vi "Fpga-FIXParser-TestHarness.vi"   [LabVIEW 2020]
uses:
  Common/Fpga-Field.Value.ctl
  <vilib>/Platform/TimedLoop/XDataNode/timing_clust.ctl
  <vilib>/Platform/TimedLoop/XDataNode/nitl_modes.ctl
  <vilib>/Platform/TimedLoop/XDataNode/wakeup.ctl
  <vilib>/rvi/Emulation/niFpgaSctlEmulationGetInTimedLoop.vi
  <vilib>/rvi/Emulation/niFpgaEmulationReportErrorSimple.vi
  <vilib>/rvi/Emulation/niFpgaGetClockAttributes.vi
  <vilib>/rvi/Emulation/niFpgaCriticalErrorInLSC.vi
  <vilib>/rvi/interface/RandomDataEmulation/niFpgaRandomDataHandleErrors.vi
  <vilib>/rvi/Emulation/niFpgaEmulationIsFPGAContextNoSignature.vi
  <vilib>/rvi/errors/niFpgaSetErrorForExecOnDevCompSimple.vi
  <vilib>/rvi/eio/common/nirviEmuReportErrorAndStop.vi
  <vilib>/rvi/DataTransferAndStorage/Container/Common/niFpgaContainerGetUniqueNameForEmu.vi
  <vilib>/rvi/FIFO/Fifo_Resource/nirvififoEmulationSetSize.vi
  <vilib>/rvi/FIFO/Fifo_Resource/nirviFifoEmulationQueueMgr.vi
  <instcachedir>/0/nirviFifoEmulationQueueMgr_E5CAEC123FF24DC58D834DCA3CDAA9B5.lvgen/nirviFifoEmulationQueueMgr_E5CAEC123FF24DC58D834DCA3CDAA9B5_002.vi
  <vilib>/rvi/FIFO/Fifo_Resource/nirvififoEmulationDetermineInputValidOut.vi
  <vilib>/rvi/FIFO/Fifo_Resource/nirvififoEmulationCreateLock.vi
  <vilib>/rvi/Emulation/niFpgaProcessEmulError.vi
  <vilib>/rvi/FIFO/Fifo_Resource/nirvififoEmulationObtainLock.vi
  <vilib>/rvi/FIFO/Fifo_Resource/nirvififoEmulationReleaseLock.vi
  <vilib>/rvi/occurrence/nirviWaitOnOccurrenceBase.vi
  <vilib>/rvi/errors/nirviReportUnexpectedCaseInternalError.vi
  <vilib>/rvi/errors/nirviReportUnexpectedCaseInternalError (U32).vi
  <instcachedir>/0/nirviFifoEmulationQueueMgr_E5CAEC123FF24DC58D834DCA3CDAA9B5.lvgen/nirviFifoEmulationQueueMgr_E5CAEC123FF24DC58D834DCA3CDAA9B5_012.vi
  <vilib>/Utility/error.llb/Clear Errors.vi
  <vilib>/Platform/TimedLoop/XDataNode/XDataNode.xnode
  <vilib>/rvi/DataTransferAndStorage/Container/XNode/niFpgaContainer.xnode
  <vilib>/rvi/interface/RandomDataEmulation/nirviRandomDataFpgaReadWriteTemplate.vi
  <vilib>/rvi/FIFO/Fifo_Resource/nirvififoEmulationWrite.vi
  <vilib>/rvi/FIFO/Fifo_Resource/nirvififoEmulationRead.vi
  <vilib>/Platform/TimedLoop/XDataNode/XDNodeRunTimeDep.lvlib
types:
  T1 = typedef "Fpga-Field.Value.ctl" = cluster{"Field.Num":u16, "Int.Value":u16, "Str.Value":u8[], "Date.Value":u64, "Str.Length":u8}
  T2 = typedef "XDNodeRunTimeDep.lvlib/timing_clust.ctl" = cluster{"Expected End [f-1]":u64, "Actual End [f-1]":u64, "Finished Late? [f-1]":bool, "Expected End [i-1]":u64, "Actual End [i-1]":u64, "Finished Late? [i-1]":bool, "Expected Start [i]":u64, "Actual Start [i]":u64, "Expected Start [f]":u64, "Actual Start [f]":u64, "Source Name":string, "Structure Name":string, "Period":i64, "Deadline":i64, "Offset":i64, "Start":i64, "Priority":i32, "Timeout":i32, "Mode":T3, "Wakeup Reason":T4, "Error":errorcluster, "Source Type":string, "Secondary Source Type":string, "Global End Time":u64, "Global Start Time":u64, "Frame Duration":u64, "Iteration Duration":u64, "Assigned CPU":i32, "I/O Scan Engine Mode":u32}
  T3 = typedef "XDNodeRunTimeDep.lvlib/nitl_modes.ctl" = enum32{"No Change", "Process missed periods, maintain original phase", "Discard missed periods, maintain original phase", "Process missed periods, ignore original phase", "Discard missed periods, ignore original phase"}
  T4 = typedef "XDNodeRunTimeDep.lvlib/wakeup.ctl" = enum32{"Normal", "Aborted", "Asynchronous wakeup", "Timing source error", "Timed loop error", "Timeout"}
  T5 = cluster{"Field.Num":u16, "Int.Value":u16, "Str.Value":u8[], "Date.Value":u64, "Str.Length":u8}
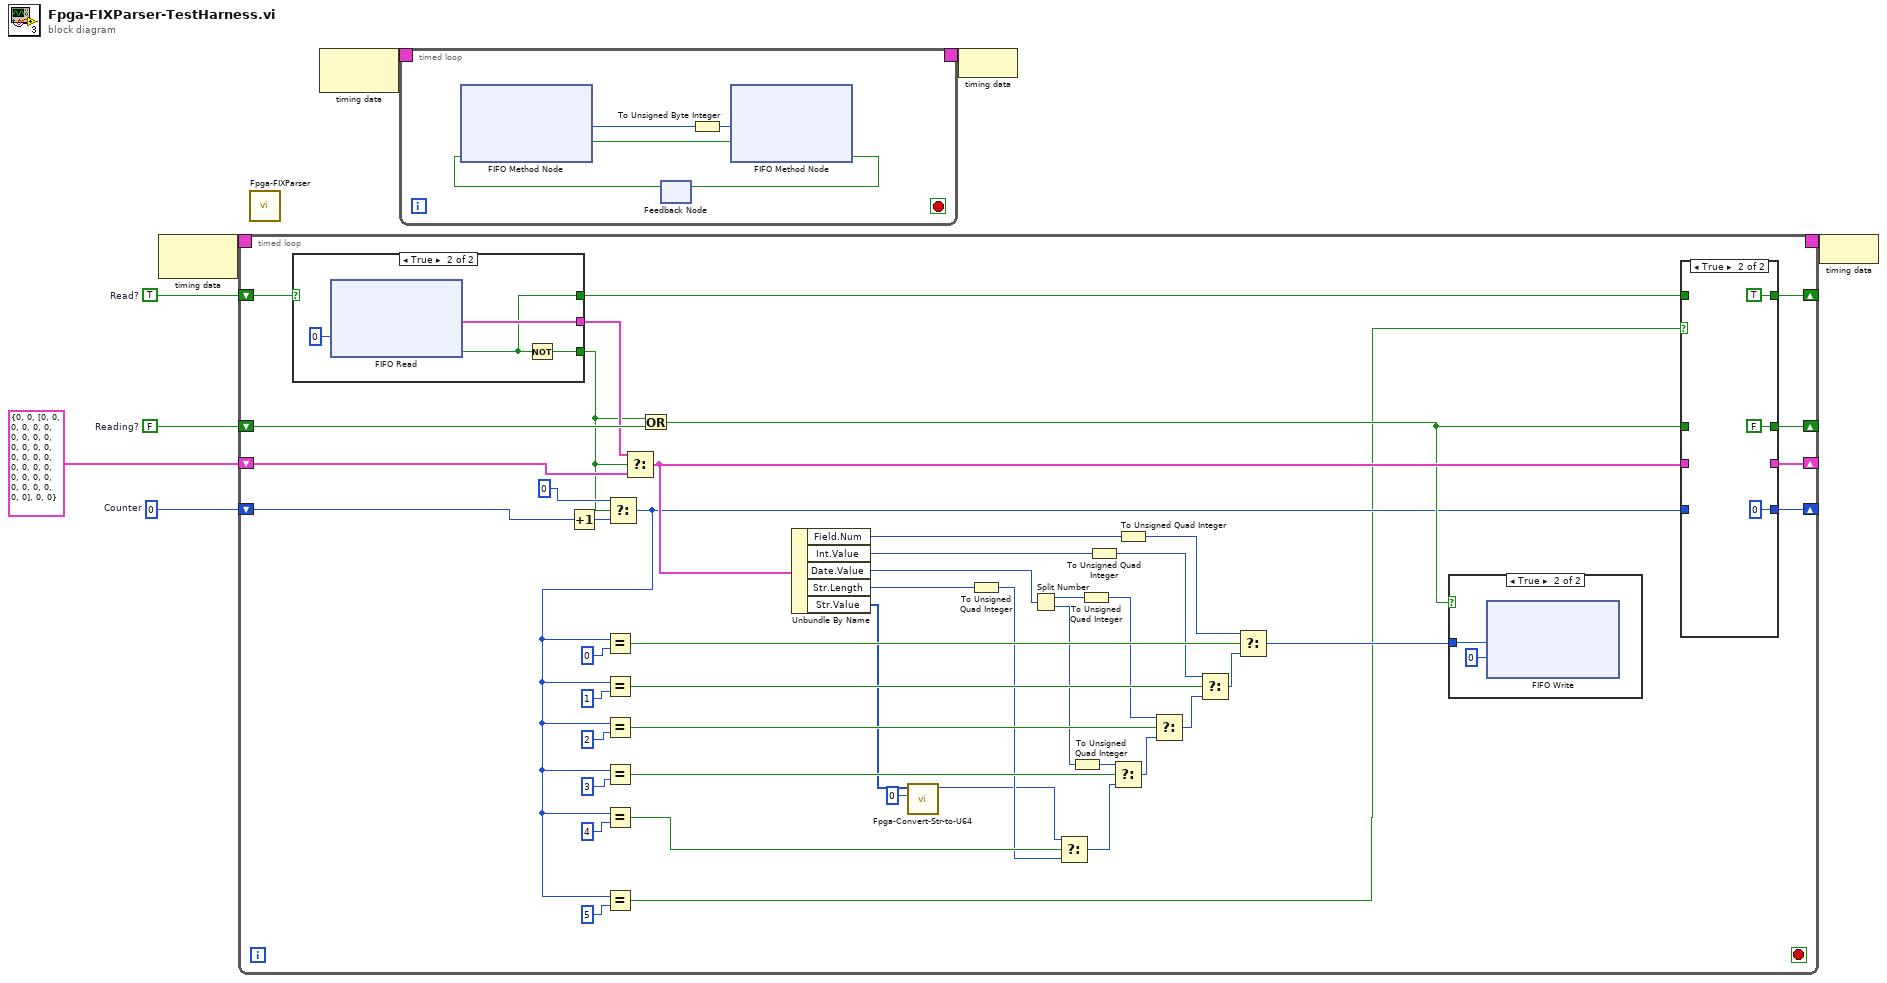
[diagram p0: block diagram]
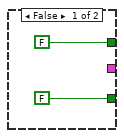
[diagram p4: hidden frame]
diagram:
  w2 = FALSE  # Reading?
  w3 = i16 0  # Counter
  w4 = TRUE  # Read?
  n1 = node-c288() -> (w6:T2)  [unwired: 1 in]
  n2 = timed-loop {
    timing: w6 -> [_]
    timing-out: [_] -> w5
    shift-right: [w53] -> _
    shift-left: w4 -> [w54]
    shift-right: [w51] -> _
    shift-left: w3 -> [w39]
    shift-right: [w49] -> _
    shift-left: w2 -> [w50]
    shift-right: [w34] -> _
    shift-left: T1 {"Field.Num"=0, "Int.Value"=0, "Str.Value"=[0, 0, 0, 0, 0, 0, 0, 0, 0, 0, 0, 0, 0, 0, 0, 0, 0, 0, 0, 0, 0, 0, 0, 0, 0, 0, 0, 0, 0, 0, 0, 0], "Date.Value"=0, "Str.Length"=0} ("Field.Value.Pair") -> [w32]
    stop <- _ stop-if-true
    n3 = case shown="True" w54 {
      tunnel: [_ w69] -> w47
      tunnel: [FALSE ("Timed Out?") w68] -> w31
      tunnel: [FALSE w67] -> w52
      frame False {
      }
      frame True {
        n4 = xnode ("FIFO Read")("Timeout"=0) -> ("Element"=w69:T5, "Timed Out?"=w67:bool)  [unwired: 1 in, 1 out]
        n5 = Not(x=w67) -> (.not. x?=w68:bool)
      }
    }
    n6 = Increment(x=w39) -> (x+1=w55:i16)
    n7 = Select(t=i16 0, s=w31, f=w55) -> (s? t:f=w17:i16)
    n8 = Equal?(x=w17, y=i16 0) -> (x = y?=w43:bool)
    n9 = Equal?(x=w17, y=i16 1) -> (x = y?=w41:bool)
    n10 = Equal?(x=w17, y=i16 2) -> (x = y?=w37:bool)
    n11 = Equal?(x=w17, y=i16 3) -> (x = y?=w21:bool)
    n12 = Equal?(x=w17, y=i16 4) -> (x = y?=w15:bool)
    n13 = Equal?(x=w17, y=i16 5) -> (x = y?=w16:bool)
    n14 = Select(t=w47, s=w31, f=w32) -> (s? t:f=w33:T1)
    n15 = Or(x=w31, y=w50) -> (x .or. y?=w30:bool)
    n16 = Unbundle By Name(w33) -> ("Field.Num"=w28:u16, "Int.Value"=w27:u16, "Date.Value"=w26:u64, "Str.Length"=w9:u8, "Str.Value"=w12:u8[])
    n17 = call "Fpga-Convert-Str-to-U64.vi"("startingIndex"=0, "Str.Value"=w12) -> ("Numeric"=w11:u64)  [unwired: 9 in]
    n18 = To Unsigned Quad Integer(1:w9) -> (0:w14:u64)
    n19 = Split Number(x=w26) -> (hi(x)=w24:u32, lo(x)=w22:u32)
    n20 = Select(t=w11, s=w15, f=w14) -> (s? t:f=w13:u64)
    n21 = To Unsigned Quad Integer(1:w22) -> (0:w19:u64)
    n22 = To Unsigned Quad Integer(1:w24) -> (0:w20:u64)
    n23 = To Unsigned Quad Integer(1:w27) -> (0:w35:u64)
    n24 = Select(t=w19, s=w21, f=w13) -> (s? t:f=w23:u64)
    n25 = To Unsigned Quad Integer(1:w28) -> (0:w36:u64)
    n26 = Select(t=w20, s=w37, f=w23) -> (s? t:f=w38:u64)
    n27 = Select(t=w35, s=w41, f=w38) -> (s? t:f=w42:u64)
    n28 = Select(t=w36, s=w43, f=w42) -> (s? t:f=w29:u64)
    n29 = case shown="True" w30 {
      tunnel: w29 -> [_ w56]
      frame False {
      }
      frame True {
        n30 = xnode ("FIFO Write")("Element"=w56, "Timeout"=0) -> ()  [unwired: 1 in, 2 out]
      }
    }
    n31 = case shown="True" w16 {
      tunnel: [w61 TRUE ("Timed Out?")] -> w53
      tunnel: w52 -> [w61 _]
      tunnel: w17 -> [w60 _]
      tunnel: [w60 i16 0 ("Counter")] -> w51
      tunnel: w30 -> [w59 _]
      tunnel: [w59 FALSE] -> w49
      tunnel: [w58 _] -> w34
      tunnel: w33 -> [w58 _]
      frame False {
      }
      frame True {
      }
    }
  }
  n32 = call "Fpga-FIXParser.vi"() -> ()  [unwired: 12 in]
  n33 = node-c288() -> (w8:T2)  [unwired: 1 in]
  n34 = timed-loop {
    timing: w8 -> [_]
    timing-out: [_] -> w7
    stop <- _ stop-if-true
    n35 = feedback #1() -> (w73:bool)  [unwired: 1 in]
    n36 = xnode ("FIFO Method Node")("Ready for Output"=w73) -> ("Element"=w77:u8, "Output Valid"=w75:bool)  [unwired: 1 in, 1 out]
    n37 = To Unsigned Byte Integer(number=w77) -> (unsigned 8bit integer=w76:u8)
    n38 = xnode ("FIFO Method Node")("Element"=w76, "Input Valid"=w75) -> ("Ready for Input"=w74:bool)  [unwired: 1 in, 1 out]
    n39 = feedback-in #1(w74) -> ()
  }
  n40 = node-c288(w7) -> ()
  n41 = node-c288(w5) -> ()
